vi "Set Offset (SubVI).vi"(2 "error in":errorcluster, 3 "Offset in":sgl, 4 "VISA Refnum in":refnum<visa-resource-name>) -> (0 "error out":errorcluster, 1 "VISA Refnum out":refnum<visa-resource-name>)   [LabVIEW 2017]
doc: "Set Offset.\nU-Link only accept 12 long string character.\nWrite the data on the COM port and check if a message is sent (to control carriage data). \nMade by Tanguy BOULARD\nTHALES FRANCE"
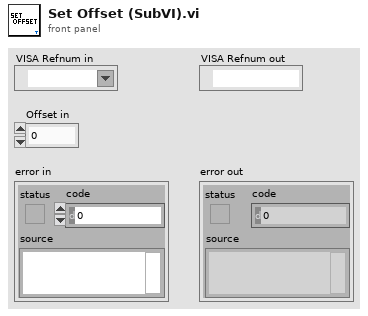
[diagram p1: front panel]
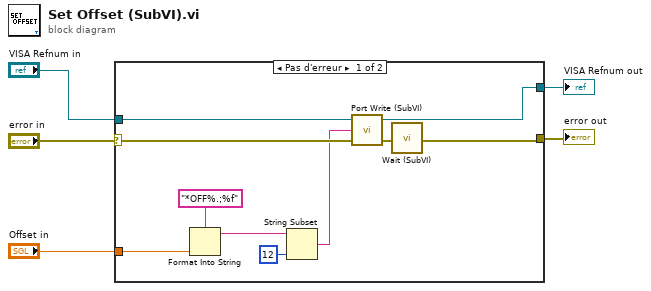
[diagram p0: block diagram]
diagram:
  n1 = case shown="Pas d'erreur" "error in" {
    selector: "error in" -> [w14 w16]
    tunnel: [w8 w16] -> w4
    tunnel: "VISA Refnum in" -> [w7 w17]
    tunnel: [w9 w17] -> w2
    tunnel: "Offset in" -> [w11 _]
    frame No Error {
      n2 = Format Into String(format string="*OFF%.;%f", w11) -> (resulting string=w13:string)  [unwired: 2 in, 1 out]
      n3 = String Subset(string=w13, length (rest)=12 ("length (rest)")) -> (substring=w6:string)  [unwired: 1 in]
      n4 = call "Port Write (SubVI).vi"("error in"=w14, "write buffer"=w6, "VISA Refnum in"=w7) -> ("error out"=w10:errorcluster, "VISA Refnum out"=w9:refnum<visa-resource-name>)  [unwired: 1 in]
      n5 = call "Wait (SubVI).vi"("error in"=w10) -> ("error out"=w8:errorcluster)  [unwired: 26 in]
    }
    frame Error {
    }
  }
  "error out" <- w4
  "VISA Refnum out" <- w2
